vi "FPGA SPI_FPGA Top Level.vi"() -> ()   [LabVIEW 2014]
uses:
  Controls/FPGA SPI_FPGA SPI State.ctl
  <vilib>/Platform/TimedLoop/XDataNode/timing_clust.ctl
  <vilib>/Platform/TimedLoop/XDataNode/nitl_modes.ctl
  <vilib>/Platform/TimedLoop/XDataNode/wakeup.ctl
  Controls/FPGA SPI_Communication Loop State.ctl
  <vilib>/rvi/Emulation/niFpgaSctlEmulationGetInTimedLoop.vi
  <vilib>/rvi/Emulation/niFpgaEmulationReportErrorSimple.vi
  <vilib>/rvi/Emulation/niFpgaGetClockAttributes.vi
  <vilib>/rvi/Emulation/niFpgaCriticalErrorInLSC.vi
  <vilib>/rvi/eio/common/nirviEmuTemplateMethod_errors.vi
  Code/FPGA SPI_Globals.vi
  <vilib>/rvi/Emulation/niFpgaProcessEmulError.vi
  <vilib>/rvi/Emulation/niFpgaEmulationIsFPGAContextNoSignature.vi
  <vilib>/rvi/errors/niFpgaSetErrorForExecOnDevCompSimple.vi
  <vilib>/rvi/eio/common/nirviEmuReportErrorAndStop.vi
  <vilib>/rvi/DataTransferAndStorage/Container/Common/niFpgaContainerGetUniqueNameForEmu.vi
  <vilib>/rvi/FIFO/Fifo_Resource/nirvififoEmulationSetSize.vi
  <vilib>/rvi/FIFO/Fifo_Resource/nirviFifoEmulationQueueMgr.vi
  <instcachedir>/0/nirviFifoEmulationQueueMgr_E5CAEC123FF24DC58D834DCA3CDAA9B5.lvgen/nirviFifoEmulationQueueMgr_E5CAEC123FF24DC58D834DCA3CDAA9B5_001.vi
  <vilib>/rvi/FIFO/Fifo_Resource/nirvififoEmulationDetermineInputValidOut.vi
  <vilib>/rvi/FIFO/Fifo_Resource/nirvififoEmulationCreateLock.vi
  <vilib>/rvi/FIFO/Fifo_Resource/nirvififoEmulationObtainLock.vi
  <vilib>/rvi/FIFO/Fifo_Resource/nirvififoEmulationReleaseLock.vi
  <vilib>/rvi/occurrence/nirviWaitOnOccurrenceBase.vi
  <vilib>/rvi/errors/nirviReportUnexpectedCaseInternalError.vi
  <vilib>/rvi/errors/nirviReportUnexpectedCaseInternalError (U32).vi
  <vilib>/Platform/TimedLoop/XDataNode/XDataNode.xnode
  <vilib>/eio/EIONode/EIONode.xnode
  <vilib>/rvi/DataTransferAndStorage/Container/XNode/niFpgaContainer.xnode
  <vilib>/rvi/FIFO/Fifo_Resource/nirvififoEmulationWrite.vi
  <vilib>/rvi/FIFO/Fifo_Resource/nirvififoEmulationRead.vi
  <vilib>/Platform/TimedLoop/XDataNode/XDNodeRunTimeDep.lvlib
panel:
  in  "CLR":bool
  in  "LDAC":bool
  in  "RESET":bool
  in  "SPI_Clock Divider":u32=20
  in  "SPI_CS Active State":bool caption="SPI_CS\nActive State"
  in  "SPI_CPOL":bool
  in  "SPI_CPHA":bool
  in  "SPI_CS":u8=1 format="%08b"
  in  "SPI_Total Bits":u16=8
  in  "SPI_Total Bytes":u16=1
  in  "SPI_Start":bool
  in  "SPI_Cmd":T1
  in  "SPI_Ack Read":bool
  out "SPI_Read Data":u8
  out "SPI_Read Flag":bool
  in  "SPI_Write Flag":bool
  in  "SPI_Write Data":u8
  in  "SPI_Port":i8
  # "Control"
  # "SPI Configuration Parameters"
  # "Command Type"
  # "Host Data Transfer"
  # "Hardware Logic Pins"
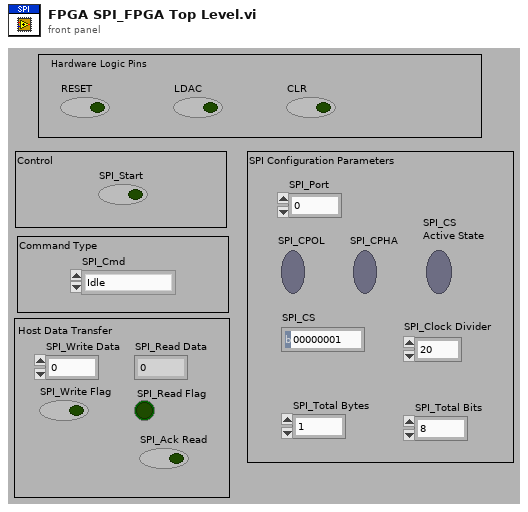
[diagram p1: front panel]
types:
  T1 = typedef "FPGA SPI_FPGA SPI State.ctl" = enum8{"Idle", "Read/Write SPI", "Configure"}
  T2 = typedef "XDNodeRunTimeDep.lvlib/timing_clust.ctl" = cluster{"Expected End [f-1]":u64, "Actual End [f-1]":u64, "Finished Late? [f-1]":bool, "Expected End [i-1]":u64, "Actual End [i-1]":u64, "Finished Late? [i-1]":bool, "Expected Start [i]":u64, "Actual Start [i]":u64, "Expected Start [f]":u64, "Actual Start [f]":u64, "Source Name":string, "Structure Name":string, "Period":i64, "Deadline":i64, "Offset":i64, "Start":i64, "Priority":i32, "Timeout":i32, "Mode":T3, "Wakeup Reason":T4, "Error":errorcluster, "Source Type":string, "Secondary Source Type":string, "Global End Time":u64, "Global Start Time":u64, "Frame Duration":u64, "Iteration Duration":u64, "Assigned CPU":i32, "I/O Scan Engine Mode":u32}
  T3 = typedef "XDNodeRunTimeDep.lvlib/nitl_modes.ctl" = enum32{"No Change", "Process missed periods, maintain original phase", "Discard missed periods, maintain original phase", "Process missed periods, ignore original phase", "Discard missed periods, ignore original phase"}
  T4 = typedef "XDNodeRunTimeDep.lvlib/wakeup.ctl" = enum32{"Normal", "Aborted", "Asynchronous wakeup", "Timing source error", "Timed loop error", "Timeout"}
  T5 = cluster{"SCLK":refnum<k21>, "CS":refnum<k21>, "MOSI":refnum<k21>, "MISO":refnum<k21>}
  T6 = typedef "FPGA SPI_Communication Loop State.ctl" = enum8{"Idle", "Init", "Write", "Start", "Read", "Wait Until Done"}
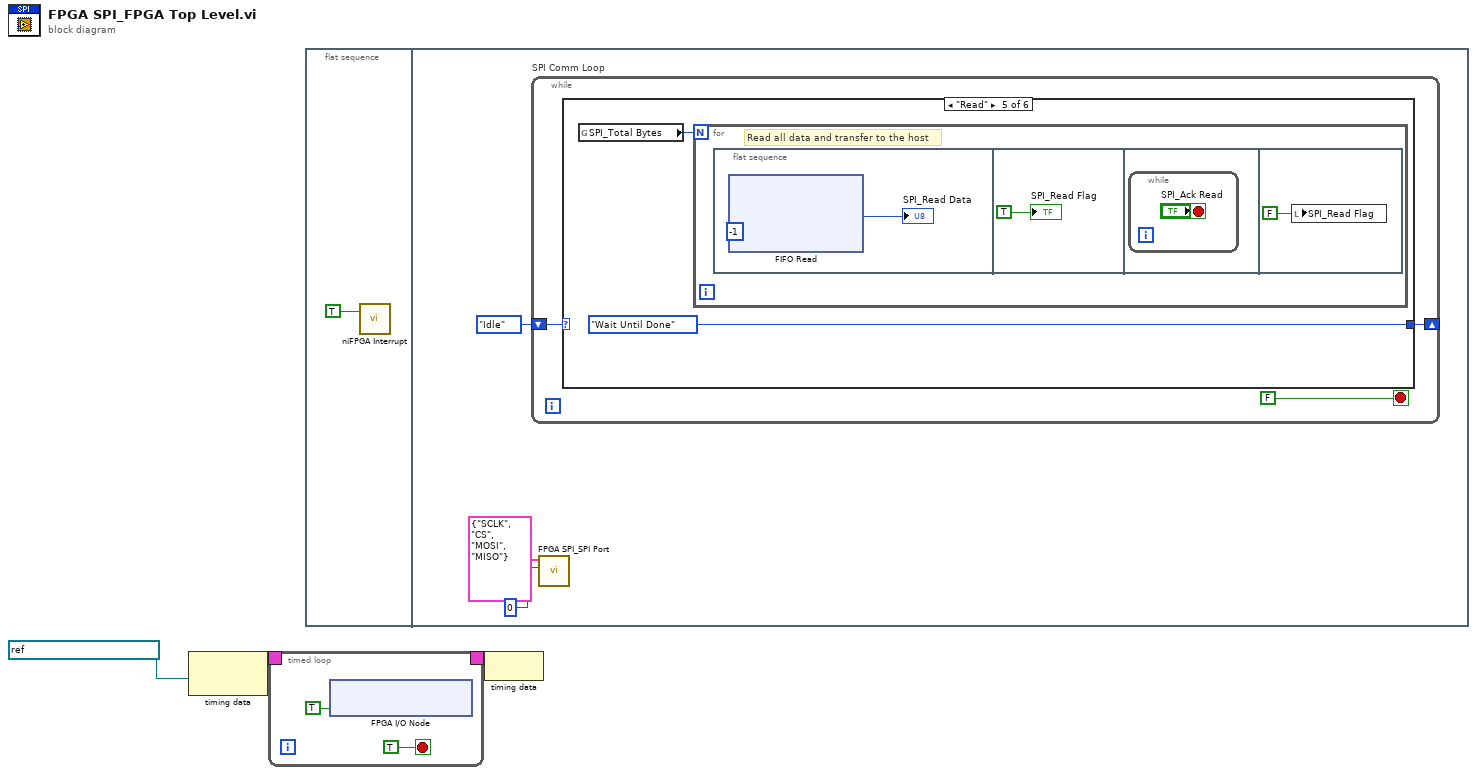
[diagram p0: block diagram]
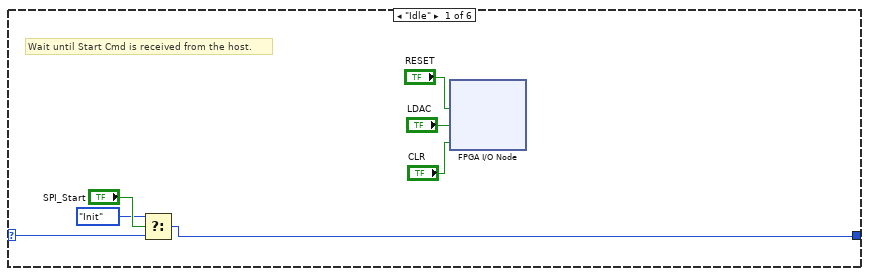
[diagram p2: hidden frame]
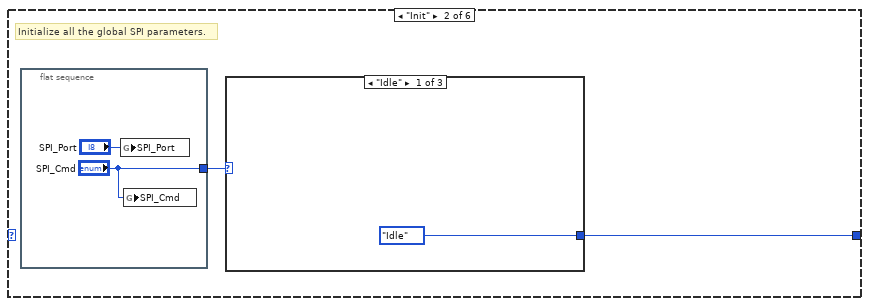
[diagram p3: hidden frame]
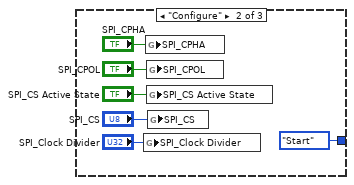
[diagram p4: hidden frame]
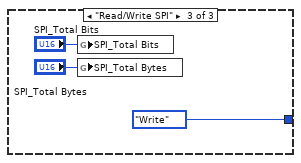
[diagram p5: hidden frame]
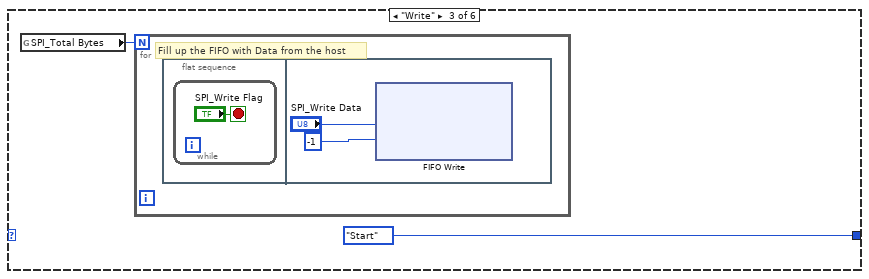
[diagram p6: hidden frame]
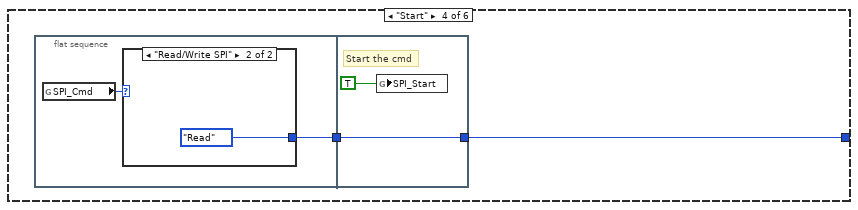
[diagram p7: hidden frame]
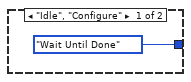
[diagram p8: hidden frame]
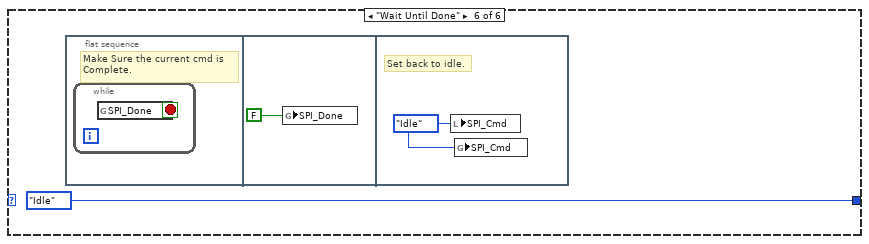
[diagram p9: hidden frame]
diagram:
  n1 = node-c288(refnum<k21> "40 MHz Onboard Clock" ("Source Name")) -> (w3:T2)
  n2 = timed-loop {
    timing: w3 -> [_]
    timing-out: [_] -> w2
    stop <- TRUE stop-if-true
    n3 = xnode "FPGA I/O Node"("Connector2/DIO29"=TRUE ("CS")) -> ()  [unwired: 1 in, 1 out]
  }
  n4 = flat-sequence {
    frame #0 {
      n5 = call <vilib>:"niFPGA Interrupt.vi"("Wait Until Cleared (F)"=TRUE ("Wait Until Cleared")) -> ()  [unwired: 2 in]
    }
    frame #1 {
      n6 = while "SPI Comm Loop" {
        shift-right: [w13] -> _
        shift-left: FPGA_SPI_Communication_Loop_State."Idle" ("Action") -> [w12]
        stop <- FALSE stop-if-true
        n7 = case shown="\"Read\"" w12 {
          selector: w12 -> [w20 _ _ _ _ _]
          tunnel: [w18 w22 FPGA_SPI_Communication_Loop_State."Start" ("Action") w42 FPGA_SPI_Communication_Loop_State."Wait Until Done" ("Action") FPGA_SPI_Communication_Loop_State."Idle" ("Action")] -> w13
          frame "Idle" {
            # "Wait until Start Cmd is received from the host."
            n8 = Select(t=FPGA_SPI_Communication_Loop_State."Init" ("Action"), s="SPI_Start", f=w20) -> (s? t:f=w18:T6)
            n9 = xnode "FPGA I/O Node"("RESET"="RESET", "LDAC"="LDAC", "CLR"="CLR") -> ()  [unwired: 3 in, 3 out]
          }
          frame "Init" {
            # "Initialize all the global SPI parameters."
            n10 = flat-sequence {
              tunnel: ["SPI_Cmd"] -> w23
              frame #0 {
                n11 = global write "FPGA SPI_Globals.vi" "SPI_Port"("SPI_Port") -> ()
                n12 = global write "FPGA SPI_Globals.vi" "SPI_Cmd"("SPI_Cmd") -> ()
              }
            }
            n13 = case shown="\"Idle\"" w23 {
              tunnel: [FPGA_SPI_Communication_Loop_State."Idle" ("Action") FPGA_SPI_Communication_Loop_State."Start" ("Action") FPGA_SPI_Communication_Loop_State."Write" ("Action")] -> w22
              frame "Idle" {
              }
              frame "Configure" {
                n14 = global write "FPGA SPI_Globals.vi" "SPI_Clock Divider"("SPI_Clock Divider") -> ()
                n15 = global write "FPGA SPI_Globals.vi" "SPI_CPHA"("SPI_CPHA") -> ()
                n16 = global write "FPGA SPI_Globals.vi" "SPI_CPOL"("SPI_CPOL") -> ()
                n17 = global write "FPGA SPI_Globals.vi" "SPI_CS Active State"("SPI_CS Active State") -> ()
                n18 = global write "FPGA SPI_Globals.vi" "SPI_CS"("SPI_CS") -> ()
              }
              frame "Read/Write SPI" {
                n19 = global write "FPGA SPI_Globals.vi" "SPI_Total Bits"("SPI_Total Bits") -> ()
                n20 = global write "FPGA SPI_Globals.vi" "SPI_Total Bytes"("SPI_Total Bytes") -> ()
              }
            }
          }
          frame "Write" {
            n21 = global read "FPGA SPI_Globals.vi" "SPI_Total Bytes"() -> (w37:u16)
            n22 = for {
              N: w37 -> [_]
              # "Fill up the FIFO with Data from the host"
              n23 = flat-sequence {
                frame #0 {
                  n24 = while {
                    stop <- "SPI_Write Flag" stop-if-true
                  }
                }
                frame #1 {
                  n25 = xnode ("FIFO Write")("Element"="SPI_Write Data", "Timeout"=-1) -> ()  [unwired: 1 in, 2 out]
                }
              }
            }
          }
          frame "Start" {
            n26 = flat-sequence {
              tunnel: [w43] -> w41
              tunnel: [w48] -> w42
              tunnel: w41 -> [w48]
              frame #0 {
                n27 = global read "FPGA SPI_Globals.vi" "SPI_Cmd"() -> (w44:T1)
                n28 = case shown="\"Read/Write SPI\"" w44 {
                  tunnel: [FPGA_SPI_Communication_Loop_State."Wait Until Done" ("Action") FPGA_SPI_Communication_Loop_State."Read" ("Action")] -> w43
                  frame "Idle", "Configure" {
                  }
                  frame "Read/Write SPI" {
                  }
                }
              }
              frame #1 {
                # "Start the cmd"
                n29 = global write "FPGA SPI_Globals.vi" "SPI_Start"(TRUE ("Write Flag")) -> ()
              }
            }
          }
          frame "Read" {
            n30 = global read "FPGA SPI_Globals.vi" "SPI_Total Bytes"() -> (w50:u16)
            n31 = for {
              N: w50 -> [_]
              # "Read all data and transfer to the host"
              n32 = flat-sequence {
                frame #0 {
                  n33 = xnode ("FIFO Read")("Timeout"=-1) -> ("Element"=→"SPI_Read Data":u8)  [unwired: 1 in, 2 out]
                }
                frame #1 {
                  "SPI_Read Flag" <- TRUE ("Read Flag")
                }
                frame #2 {
                  n34 = while {
                    stop <- "SPI_Ack Read" stop-if-true
                  }
                }
                frame #3 {
                  n35 = local write "SPI_Read Flag"(FALSE ("Read Flag")) -> ()
                }
              }
            }
          }
          frame "Wait Until Done" {
            n36 = flat-sequence {
              frame #0 {
                # "Make Sure the current cmd is\nComplete."
                n37 = while {
                  stop <- w57 stop-if-true
                  n38 = global read "FPGA SPI_Globals.vi" "SPI_Done"() -> (w57:bool)
                }
              }
              frame #1 {
                n39 = global write "FPGA SPI_Globals.vi" "SPI_Done"(FALSE ("Done")) -> ()
              }
              frame #2 {
                w59 = FPGA_SPI_FPGA_SPI_State."Idle" ("Type")
                # "Set back to idle."
                n40 = local write "SPI_Cmd"(w59) -> ()
                n41 = global write "FPGA SPI_Globals.vi" "SPI_Cmd"(w59) -> ()
              }
            }
          }
        }
      }
      n42 = call "FPGA SPI_SPI Port.vi"("Port"=i8 0, "FPGA IO"=T5 {"SCLK"="SCLK", "CS"="CS", "MOSI"="MOSI", "MISO"="MISO"}) -> ()  [unwired: 10 out]
    }
  }
  n43 = node-c288(w2) -> ()
